vi "Control Hilight Display(冲突时的文件备份2013-05-03 10-27-40).vi"(8 "错误输入（无错误）":errorcluster, 11 "Ctl Ref In":refnum<vi>) -> (0 "错误输出":errorcluster, 3 "Ctl Ref Out":refnum<vi>)   [LabVIEW 2012, in "CtrlRef.lvlib"]
uses:
  CtrlRef.lvlib
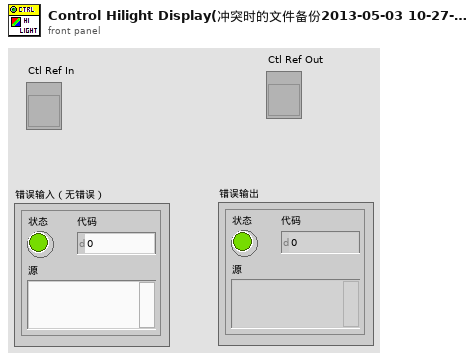
[diagram p1: front panel]
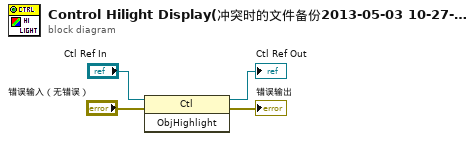
[diagram p0: block diagram]
diagram:
  n1 = invoke class="Ctl" method="ObjHighlight"(reference="Ctl Ref In", error in="错误输入（无错误）") -> (reference out=→"Ctl Ref Out":refnum<vi>, error out=→"错误输出":errorcluster)  [unwired: 1 in, 1 out]
